vi "Update Progress.vi"(8 "error in (no error)":errorcluster, 9 "Troubleshoot?":bool, 10 "User State":T7=enum."Deploy", 11 "Ctl Refs in":T1) -> (0 "error out":errorcluster, 3 "Ctl Refs out":T1)   [LabVIEW 2013]
uses:
  types/UserStateType.ctl
  Controls/Refs.ctl
  Controls/Button Refs.ctl
  Controls/Tab Ctl Refs.ctl
  types/TabStateType.ctl
  Controls/Indicator Refs.ctl
  Controls/Slider Refs.ctl
  Controls/Control Refs.ctl
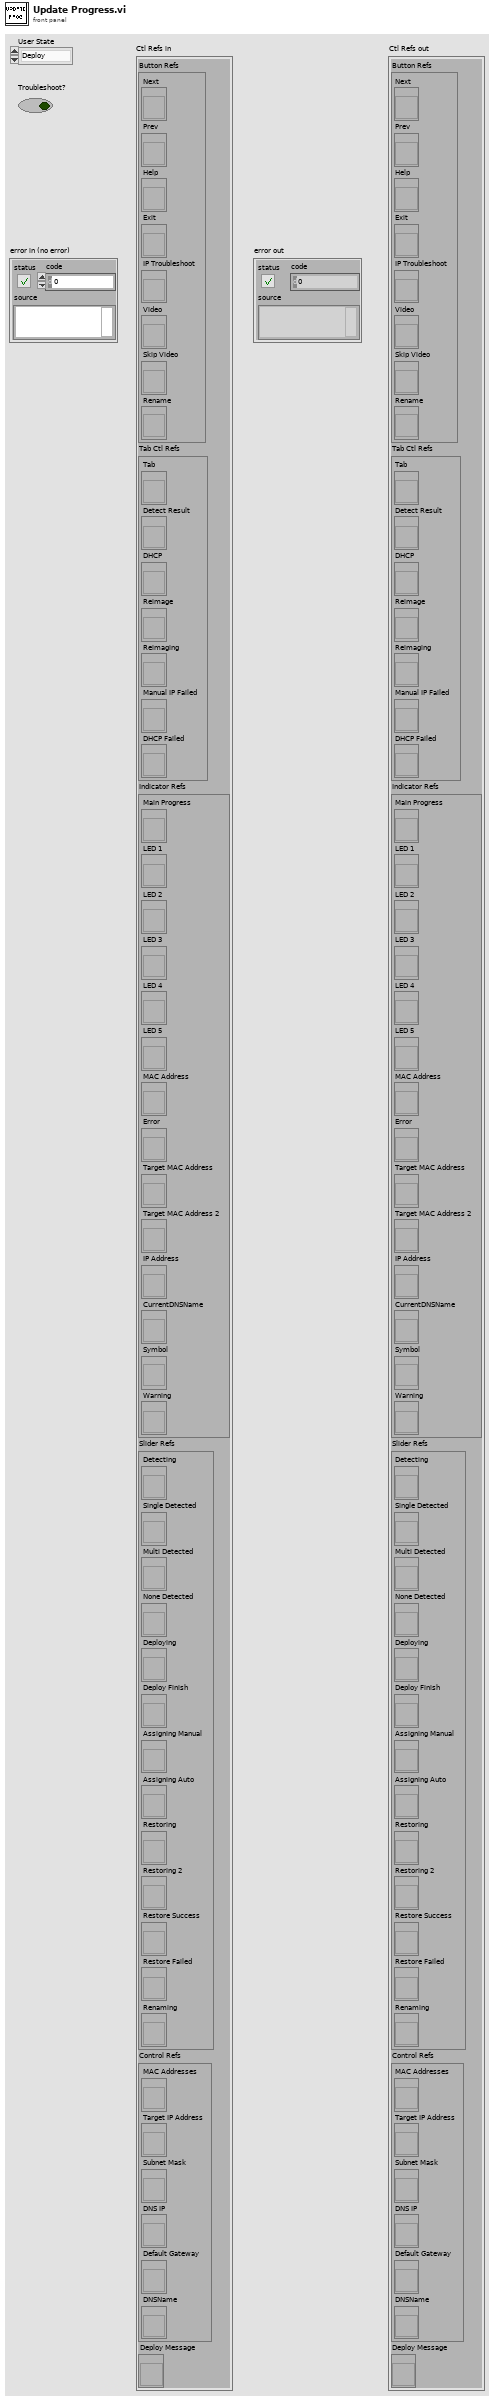
[diagram p1: front panel]
types:
  T1 = typedef "Refs.ctl" = cluster{"Button Refs":T2, "Tab Ctl Refs":T3, "Indicator Refs":T4, "Slider Refs":T5, "Control Refs":T6, "Deploy Message":refnum<vi>}
  T2 = typedef "Button Refs.ctl" = cluster{"Next":refnum<vi>, "Prev":refnum<vi>, "Help":refnum<vi>, "Exit":refnum<vi>, "IP Troubleshoot":refnum<vi>, "Video":refnum<vi>, "Skip Video":refnum<vi>, "Rename":refnum<vi>}
  T3 = typedef "Tab Ctl Refs.ctl" = cluster{"Tab":refnum<vi>, "Detect Result":refnum<vi>, "DHCP":refnum<vi>, "Reimage":refnum<vi>, "Reimaging":refnum<vi>, "Manual IP Failed":refnum<vi>, "DHCP Failed":refnum<vi>}
  T4 = typedef "Indicator Refs.ctl" = cluster{"Main Progress":refnum<vi>, "LED 1":refnum<vi>, "LED 2":refnum<vi>, "LED 3":refnum<vi>, "LED 4":refnum<vi>, "LED 5":refnum<vi>, "MAC Address":refnum<vi>, "Error":refnum<vi>, "Target MAC Address":refnum<vi>, "Target MAC Address 2":refnum<vi>, "IP Address":refnum<vi>, "CurrentDNSName":refnum<vi>, "Symbol":refnum<vi>, "Warning":refnum<vi>}
  T5 = typedef "Slider Refs.ctl" = cluster{"Detecting":refnum<vi>, "Single Detected":refnum<vi>, "Multi Detected":refnum<vi>, "None Detected":refnum<vi>, "Deploying":refnum<vi>, "Deploy Finish":refnum<vi>, "Assigning Manual":refnum<vi>, "Assigning Auto":refnum<vi>, "Restoring":refnum<vi>, "Restoring 2":refnum<vi>, "Restore Success":refnum<vi>, "Restore Failed":refnum<vi>, "Renaming":refnum<vi>}
  T6 = typedef "Control Refs.ctl" = cluster{"MAC Addresses":refnum<vi>, "Target IP Address":refnum<vi>, "Subnet Mask":refnum<vi>, "DNS IP":refnum<vi>, "Default Gateway":refnum<vi>, "DNSName":refnum<vi>}
  T7 = typedef "UserStateType.ctl" = enum16{"Welcome", "Instructions", "Detect", "Deploy", "Success"}
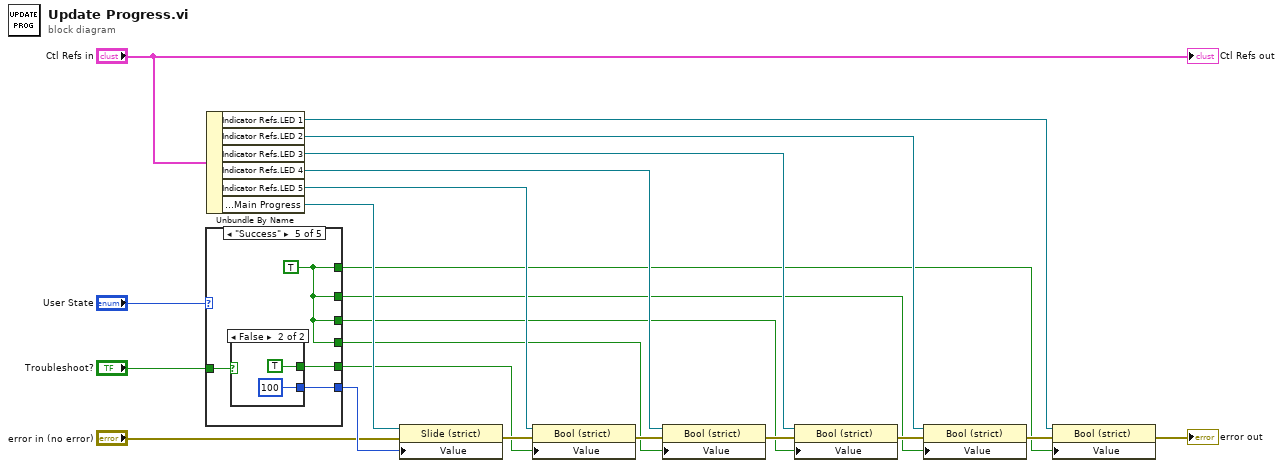
[diagram p0: block diagram]
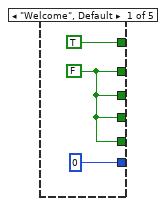
[diagram p2: hidden frame]
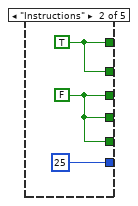
[diagram p3: hidden frame]
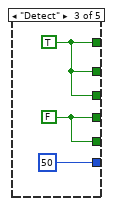
[diagram p4: hidden frame]
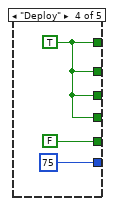
[diagram p5: hidden frame]
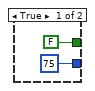
[diagram p6: hidden frame]
diagram:
  n1 = case shown="\"Success\"" "User State" {
    tunnel: [TRUE w27 w29 w32 w36] -> w3
    tunnel: [w24 w27 w29 w32 w36] -> w4
    tunnel: [w24 w26 w29 w32 w36] -> w5
    tunnel: [w24 w26 w30 w32 w36] -> w6
    tunnel: [w24 w26 w30 FALSE w37] -> w7
    tunnel: [u8 0 ("Main Progress") u8 25 ("Main Progress") u8 50 ("Main Progress") u8 75 ("Main Progress") w38] -> w8
    tunnel: "Troubleshoot?" -> [_ _ _ _ w35]
    frame "Welcome", Default {
      w24 = FALSE
    }
    frame "Instructions" {
      w26 = FALSE
      w27 = TRUE
    }
    frame "Detect" {
      w30 = FALSE
      w29 = TRUE
    }
    frame "Deploy" {
      w32 = TRUE
    }
    frame "Success" {
      w36 = TRUE
      n2 = case shown="False" w35 {
        tunnel: [u8 75 ("Main Progress") u8 100 ("Main Progress")] -> w38
        tunnel: [FALSE TRUE] -> w37
        frame True {
        }
        frame False {
        }
      }
    }
  }
  n3 = Unbundle By Name("Ctl Refs in") -> ("Indicator Refs.LED 1"=w14:refnum<vi>, "Indicator Refs.LED 2"=w15:refnum<vi>, "Indicator Refs.LED 3"=w16:refnum<vi>, "Indicator Refs.LED 4"=w17:refnum<vi>, "Indicator Refs.LED 5"=w18:refnum<vi>, "Indicator Refs.Main Progress"=w20:refnum<vi>)
  n4 = property class="Slide (strict)"(reference=w20, error in="error in (no error)", "Value"=w8) -> (error out=w19:errorcluster)  [unwired: 1 out]
  n5 = property class="Bool (strict)"(reference=w18, error in=w19, "Value"=w7) -> (error out=w10:errorcluster)  [unwired: 1 out]
  n6 = property class="Bool (strict)"(reference=w17, error in=w10, "Value"=w6) -> (error out=w11:errorcluster)  [unwired: 1 out]
  n7 = property class="Bool (strict)"(reference=w16, error in=w11, "Value"=w5) -> (error out=w12:errorcluster)  [unwired: 1 out]
  n8 = property class="Bool (strict)"(reference=w15, error in=w12, "Value"=w4) -> (error out=w13:errorcluster)  [unwired: 1 out]
  n9 = property class="Bool (strict)"(reference=w14, error in=w13, "Value"=w3) -> (error out=→"error out":errorcluster)  [unwired: 1 out]
  "Ctl Refs out" <- "Ctl Refs in"
